vi "Send frame rate.vi"(8 "error in (no error)":errorcluster, 11 "DAQOrcaFlash in":refnum<class "DAQOrcaFlash.lvclass">) -> (0 "error out":errorcluster, 3 "DAQOrcaFlash out":refnum<class "DAQOrcaFlash.lvclass">)   [LabVIEW 2012, in "DAQOrcaFlash.lvclass"]
uses:
  DAQOrcaFlash.lvclass
  <vilib>/Distrio/Murmex/Murmex/update_cluster.ctl
  DAQOrcaFlash.lvclass/DAQOrcaFlash.ctl
  <vilib>/Distrio/Murmex/Murmex/Murmex.lvclass
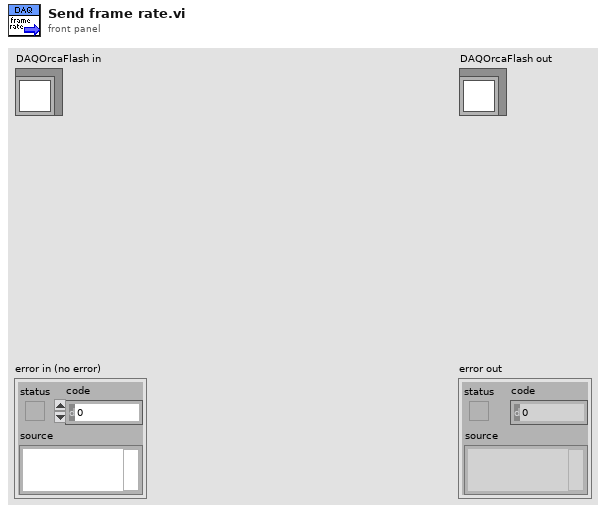
[diagram p1: front panel]
types:
  T1 = typedef "Murmex.lvlib/Murmex.lvclass/update_cluster.ctl" = cluster{"target ID":string, "key chains":string[], "values":variant[]}
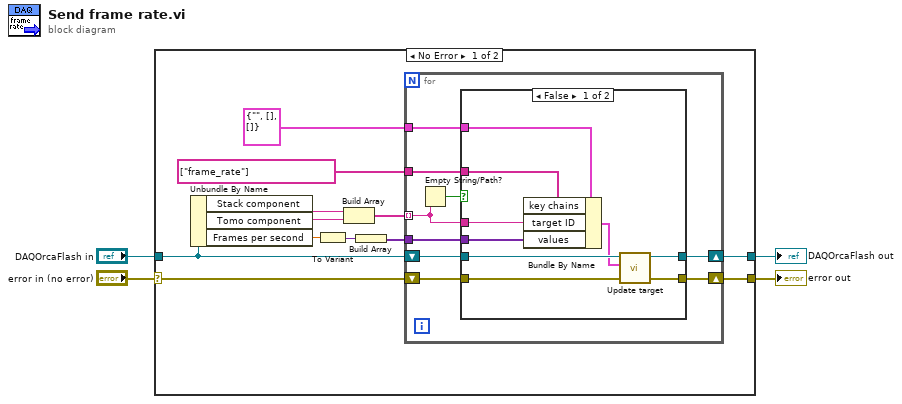
[diagram p0: block diagram]
diagram:
  n1 = case shown="No Error" "error in (no error)" {
    selector: "error in (no error)" -> [w16 w37]
    tunnel: [w15 w37] -> w1
    tunnel: [w13 w38] -> w2
    tunnel: "DAQOrcaFlash in" -> [w14 w38]
    frame No Error {
      n2 = Unbundle By Name(w14) -> ("Stack component"=w8:string, "Tomo component"=w9:string, "Frames per second"=w12:dbl[unit])
      n3 = To Variant(anything=w12) -> (Variant=w11:variant)
      n4 = Build Array(w8, w9) -> (w7:string[])
      n5 = Build Array(w11) -> (w10:variant[])
      n6 = for {
        tunnel: w10 -> [w21]
        tunnel: w7 -> [w18] mode=indexing
        tunnel: string[] ["frame_rate"] ("key chains") -> [w20]
        tunnel: T1 {"target ID"="", "key chains"=[], "values"=[]} ("update cluster") -> [w19]
        shift-right: [w24] -> w15
        shift-left: w16 -> [w25]
        shift-right: [w22] -> w13
        shift-left: w14 -> [w23]
        n7 = Empty String/Path?(string/path=w18) -> (empty?=w17:bool)
        n8 = case shown="False" w17 {
          tunnel: w25 -> [w34 w35]
          tunnel: [w33 w35] -> w24
          tunnel: w23 -> [w32 w36]
          tunnel: [w31 w36] -> w22
          tunnel: w21 -> [w30 _]
          tunnel: w20 -> [w29 _]
          tunnel: w19 -> [w28 _]
          tunnel: w18 -> [w26 _]
          frame False {
            n9 = Bundle By Name(cluster=w28, "key chains"=w29, "target ID"=w26, "values"=w30) -> (w27:T1)
            n10 = call <vilib>:"Update target.vi"("error in (no error)"=w34, "update cluster"=w27, "MurmexBase in"=w32) -> ("error out"=w33:errorcluster, "MurmexBase out"=w31:refnum<class "DAQOrcaFlash.lvclass">)  [unwired: 7 in]
          }
          frame True {
          }
        }
      }
    }
    frame Error {
    }
  }
  "error out" <- w1
  "DAQOrcaFlash out" <- w2
